vi "NeuronID_UDP_send_v008.vi"(2 "error in (no error)":errorcluster, 3 "Neuron ID":dbl(slide) scale=0.0..10.0, 5 "UDP Network Connection in":refnum<k16>) -> (0 "error out":errorcluster, 1 "UDP Network Connection out":refnum<k16>)   [LabVIEW 2019]
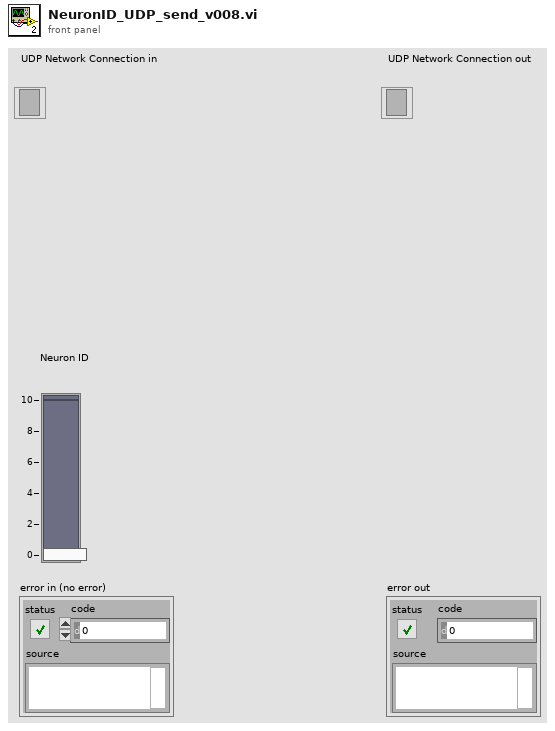
[diagram p1: front panel]
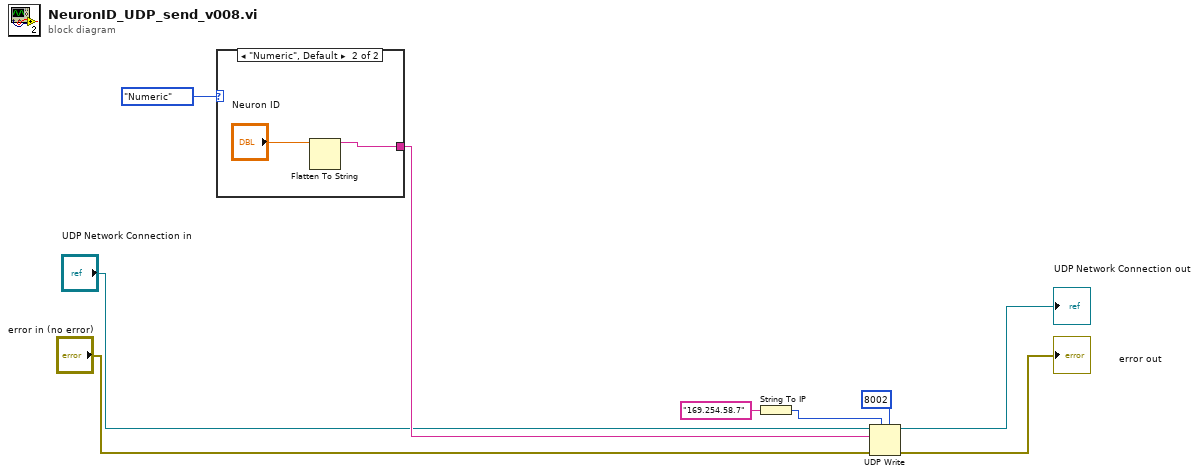
[diagram p0: block diagram]
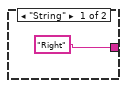
[diagram p2: hidden frame]
diagram:
  n1 = case shown="\"Numeric\", Default" enum16{"String", "Numeric"}."Numeric" ("Data to send") {
    tunnel: ["Right" ("Message") w12] -> w7
    frame "String" {
    }
    frame "Numeric", Default {
      n2 = Flatten To String(anything="Neuron ID") -> (data string=w12:string)  [unwired: 3 in, 2 out]
    }
  }
  n3 = String To IP(1:"169.254.58.7" ("name")) -> (0:w2:u32)
  n4 = UDP Write(address=w2, port or service name=u16 8002, connection ID="UDP Network Connection in", data in=w7, 8:"error in (no error)") -> (error out=→"error out":errorcluster, 3:→"UDP Network Connection out":refnum<k16>)  [unwired: 1 in]
